vi "PH_ImageCoG_Plotter.check Cam Settings.vi"(0 "i ref in":refnum<vi>, 5 "error out":errorcluster) -> (14 "i ref out":refnum<vi>, 19 "error out":errorcluster)   [LabVIEW 2014, in "PH_ImageCoG_Plotter.lvlib"]
doc: "This VI checks whether the current cam settings are the same as stored in the calibration data. It sets the related GUI elements and own attributes."
uses:
  PH_ImageCoG_Plotter.lvlib
  PH_Basics/PH_StatusHandler/PH_StatusHandler.Status.ctl
  PH_Basics/PH_Common/PH_Common.lvlib
  PH_Basics/PH_Img_BaseClass/PH_Img_BaseClass.lvlib
  PH_Basics/PH_StatusHandler/PH_StatusHandler.lvlib
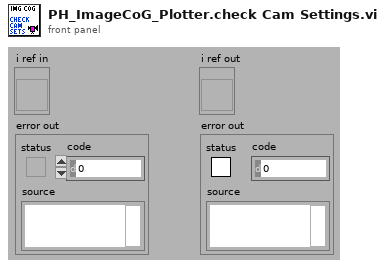
[diagram p1: front panel]
types:
  T1 = typedef "PH_StatusHandler.lvlib/PH_StatusHandler.Status.ctl" = i16
  T2 = typedef "PH_ImageCoG_Plotter.lvlib/PH_ImageCoG_Plotter.i attribute.ctl" = cluster{"GUI Refs":cluster{"Delete":refnum<vi>, "Calibration status":refnum<vi>, "BI subtracted":refnum<vi>, "calc Beam Anal":refnum<vi>, "CoG - x":refnum<vi>, "CoG - y":refnum<vi>, "Type":refnum<vi>, "Center":refnum<vi>, "exp - X":refnum<vi>, "exp - Y":refnum<vi>, "Delta - X":refnum<vi>, "Delta - Y":refnum<vi>, "Available Cams":refnum<vi>, "CoG X":refnum<vi>, "CoG Y":refnum<vi>, "Delta X":refnum<vi>, "Delta Y":refnum<vi>, "Export Data":refnum<vi>, "Calibration data":refnum<vi>}, "Calibration":cluster{"Status":T1, "Calibration data":T3, "Calibration Data File":path}, "Beam Analysis":cluster{"on":bool, "exp - X":i32, "exp - Y":i32, "Type":bool, "Data":cluster{"current time":timestamp, "CoG-x":dbl, "CoG-y":dbl, "Delta-x":dbl, "Delta-y":dbl}[], "Datasets strored":i32, "Dataarray Size":i32}, "Cam instances":string[], "DIM Service Events":T4[], "Images":cluster{"Background":T7, "OP":T7, "GUI":T7}}
  T3 = typedef "PH_ImageCalibrator.lvlib/PH_ImageCalibrator.Calibration Data.ctl" = cluster{"Date":string, "Time":string, "Cam Settings":cluster{"Cam ID":string, "Gain":dbl, "Brightness":dbl, "Shutter":dbl, "Cam Error":bool, "Mode":i32}, "Background Image":cluster{"Image":dbl[][], "Image Error":bool}, "Linear Calibration":cluster{"Calibration Factor":dbl, "not mm or mrad":bool}, "Energy Calibration":cluster{"Calibration Factor":dbl, "no mJ":bool}}
  T4 = typedef "BaseProcess.lvlib/BaseProcess.event definition.ctl" = cluster{"CAEEvtDef":T5, "Data Descriptor":T6}
  T5 = typedef "CAEObj.lvlib/CAEObj.event definition.ctl" = cluster{"URL":string, "enable":bool, "ignoreResID":bool}
  T6 = typedef "BaseProcess.lvlib/BaseProcess.descriptor string definition.ctl" = string
  T7 = typedef "IMAQ Image.ctl" = refnum<image>
  T8 = cluster{"Cam ID":string, "Gain":dbl, "Brightness":dbl, "Shutter":dbl, "Cam Error":bool, "Mode":i32}
  T9 = typedef "PH_Img_BaseClass.lvlib/PH_Img_BaseClass.i attribute.ctl" = cluster{"GUI Refs":T10, "Timeout Image [ms]":i32, "Default Periodic Period [ms]":i32, "Camera":cluster{"Instancename":string, "Notifier":refnum<notifier>}, "Palette":T11, "Cam Settings":cluster{"Cam ID":string, "Gain":dbl, "Brightness":dbl, "Shutter":dbl, "Cam Info Failure":bool, "Mode":i32}}
  T10 = typedef "PH_Img_BaseClass.lvlib/PH_Img_BaseClass.GUI Refs.ctl" = cluster{"Timeout":refnum<vi>, "Image":refnum<vi>, "Palette":refnum<vi>, "Timeout Set":refnum<vi>}
  T11 = typedef "PH_Img_BaseClass.lvlib/PH_Img_BaseClass.Palette.ctl" = i32
  T12 = cluster{"Cam ID":string, "Gain":dbl, "Brightness":dbl, "Shutter":dbl, "Cam Info Failure":bool, "Mode":i32}
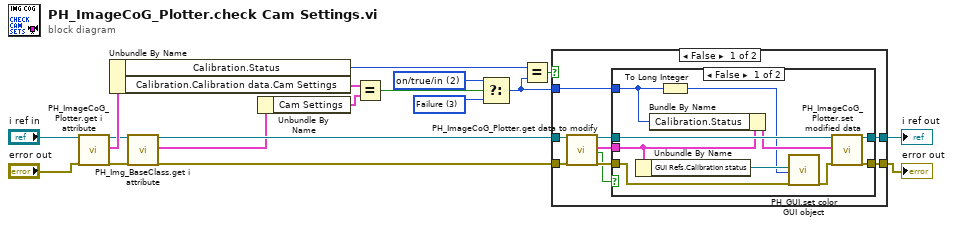
[diagram p0: block diagram]
diagram:
  w13 = T1 2 items=["no info", "off/false/out", "on/true/in", "Failure", "Alarm", "Status 1", "Status 2", "Status 3"] ("Calibration.Status")
  w12 = T1 3 items=["no info", "off/false/out", "on/true/in", "Failure", "Alarm", "Status 1", "Status 2", "Status 3"] ("Calibration.Status")
  n1 = call "PH_ImageCoG_Plotter.get i attribute.vi"("i ref in"="i ref in", "error in (no error)"="error out") -> ("i ref out"=w4:refnum<vi>, "i attribute"=w16:T2, "error out"=w6:errorcluster)  [unwired: 15 in]
  n2 = Unbundle By Name(w16) -> ("Calibration.Status"=w14:T1, "Calibration.Calibration data.Cam Settings"=w15:T8)
  n3 = call "PH_Img_BaseClass.get i attribute.vi"("i ref in"=w4, "error in (no error)"=w6) -> ("i ref out"=w3:refnum<vi>, "i attribute"=w2:T9, "error out"=w5:errorcluster)  [unwired: 15 in]
  n4 = Unbundle By Name(w2) -> ("Cam Settings"=w1:T12)
  n5 = Equal?(x=w15, y=w1) -> (x = y?=w7:bool)
  n6 = Select(t=w13, s=w7, f=w12) -> (s? t:f=w10:T1)
  n7 = Equal?(x=w14, y=w10) -> (x = y?=w11:bool)
  n8 = case shown="False" w11 {
    tunnel: w5 -> [w25 w40]
    tunnel: [w24 w40] -> w9
    tunnel: w3 -> [w23 w41]
    tunnel: [w22 w41] -> w8
    tunnel: w10 -> [w20 _]
    frame False {
      n9 = call "PH_ImageCoG_Plotter.get data to modify.vi"("i ref in"=w23, "error in (no error)"=w25) -> ("i ref out"=w27:refnum<vi>, "i attribute"=w21:T2, "timed out"=w19:bool, "error out"=w26:errorcluster)  [unwired: 14 in]
      n10 = case shown="False" w19 {
        tunnel: w27 -> [w37 w39]
        tunnel: w26 -> [w29 w38]
        tunnel: [w36 w38] -> w24
        tunnel: [w35 w39] -> w22
        tunnel: w21 -> [w33 _]
        tunnel: w20 -> [w30 _]
        frame False {
          n11 = Unbundle By Name(w33) -> ("GUI Refs.Calibration status"=w31:refnum<vi>)
          n12 = Bundle By Name(cluster=w33, "Calibration.Status"=w30) -> (w34:T2)
          n13 = To Long Integer(number=w30) -> (32bit integer=w28:i32)
          n14 = call "PH_GUI.set color GUI object.vi"("GUI object Ref"=w31, "State"=w28, "error in (no error)"=w29) -> ("error out"=w32:errorcluster)  [unwired: 16 in]
          n15 = call "PH_ImageCoG_Plotter.set modified data.vi"("i ref in"=w37, "i attribute"=w34, "error in (no error)"=w32) -> ("i ref out"=w35:refnum<vi>, "error out"=w36:errorcluster)  [unwired: 15 in]
        }
        frame True {
        }
      }
    }
    frame True {
    }
  }
  "error out" <- w9
  "i ref out" <- w8
